vi "get_pico_rapid_data.vi"(8 "error in":errorcluster, 11 "PicoScope Acquisition Settings":T1={"Channel A Settings"={"Enabled"=TRUE, "Coupling"=1, "Range"=6, "Analogue Offset"=0.0}, "Channel B Settings"={"Enabled"=TRUE, "Coupling"=1, "Range"=6, "Analogue Offset"=0.0}, "Trigger Options"={"Trigger Enabled"=FALSE, "Trigger Source"=enum."Channel A", "Trigger Threshold (-5 to 5 V)"=0.0, "Trigger Slope"=2, "Trigger Delay (s)"=0.0, "Auto Trigger Time (ms)"=1000}, "Pico Scope Inititalization Settings"={"USB Power"=FALSE, "Use Serial Number"=FALSE, "Resolution"=0, "Serial Number"="", "Handle"=0}, "Use PicoScope?"=FALSE, "Acquisition Settings"={"Pre Trigger Time (s)"=512.0, "Post Trigger Time (s)"=512.0, "Resolution (s)"=34.36, "Four Channel Device"=FALSE, "Number of Captures"=1.0}} {"Acquisition Settings"."Number of Captures" min=1.0 step=1.0; "Acquisition Settings"."Resolution (s)" min=8e-09 max=34.36 step=8e-09 format="%#_6p"; "Acquisition Settings"."Post Trigger Time (s)" min=0.0 format="%#_6p"; "Acquisition Settings"."Pre Trigger Time (s)" min=0.0 format="%#_6p"; "Pico Scope Inititalization Settings"."Resolution" items=["8-bit", "12-bit", "14-bit", "15-bit (max. 2 ch.)", "16-bit (max. 1 ch.)"]; "Trigger Options"."Trigger Slope" items=["Rising"=2, "Falling"=3]; "Channel B Settings"."Range" items=["10 mV", "20 mV", "50 mV", "100 mV", "200 mV", "500 mV", "1 V", "2 V", "5 V", "10 V", "20 V", "50 V ", "100 V"]; "Channel B Settings"."Coupling" items=["AC", "DC"]; "Channel A Settings"."Range" items=["10 mV", "20 mV", "50 mV", "100 mV", "200 mV", "500 mV", "1 V", "2 V", "5 V", "10 V", "20 V", "50 V ", "100 V"]; "Channel A Settings"."Coupling" items=["AC", "DC"]}) -> (0 "error out":errorcluster, 2 "Channel B Out":dbl[][][](array[numeric]), 3 "Channel A Out":dbl[][][](array[numeric]))   [LabVIEW 2016]
uses:
  Controls/PicoScope/pico_control_panel.ctl
  Controls/PicoScope/pico_channel_settings.ctl
  Controls/PicoScope/pico_trigger.ctl
  Controls/PicoScope/pico_init_settings.ctl
panel:
  out "size(s)":i32[](array[numeric])
  out "Channel A Buffer":i16[][](array[numeric])
  out "Channel B Buffer":i16[][](array[numeric])
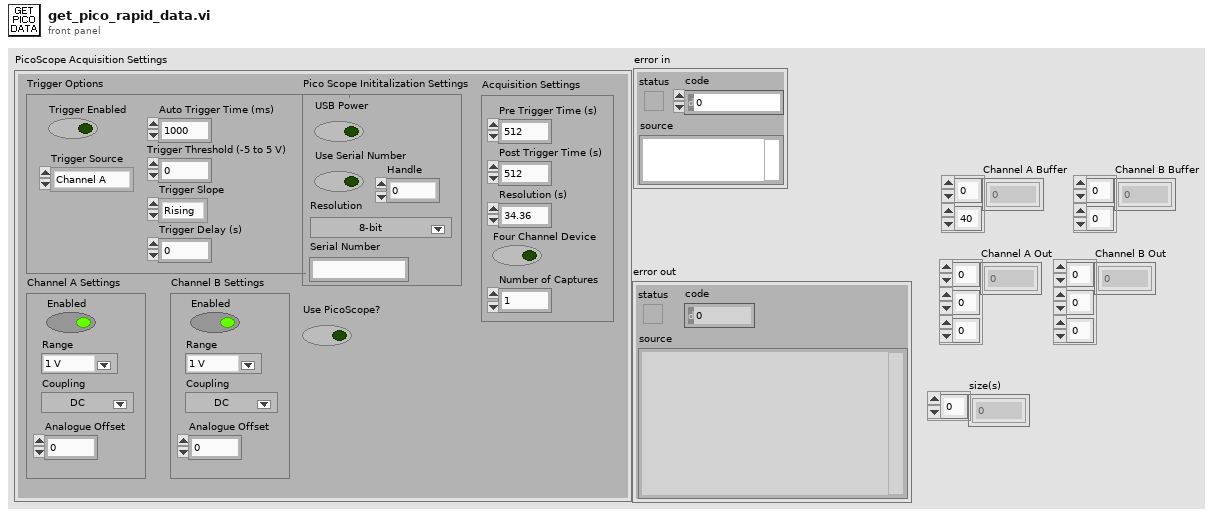
[diagram p1: front panel]
types:
  T1 = typedef "pico_control_panel.ctl" = cluster{"Channel A Settings":T2, "Channel B Settings":T2, "Trigger Options":T3, "Pico Scope Inititalization Settings":T4, "Use PicoScope?":bool, "Acquisition Settings":cluster{"Pre Trigger Time (s)":dbl, "Post Trigger Time (s)":dbl, "Resolution (s)":dbl, "Four Channel Device":bool, "Number of Captures":dbl}}
  T2 = typedef "pico_channel_settings.ctl" = cluster{"Enabled":bool, "Coupling":i16, "Range":u16, "Analogue Offset":sgl}
  T3 = typedef "pico_trigger.ctl" = cluster{"Trigger Enabled":bool, "Trigger Source":enum16{"Channel A", "Channel B", "Channel C", "Channel D", "Ext."}, "Trigger Threshold (-5 to 5 V)":dbl, "Trigger Slope":u16, "Trigger Delay (s)":dbl, "Auto Trigger Time (ms)":i16}
  T4 = typedef "pico_init_settings.ctl" = cluster{"USB Power":bool, "Use Serial Number":bool, "Resolution":i32, "Serial Number":string, "Handle":i16}
  T5 = cluster{"Pre Trigger Time (s)":dbl, "Post Trigger Time (s)":dbl, "Resolution (s)":dbl, "Four Channel Device":bool, "Number of Captures":dbl}
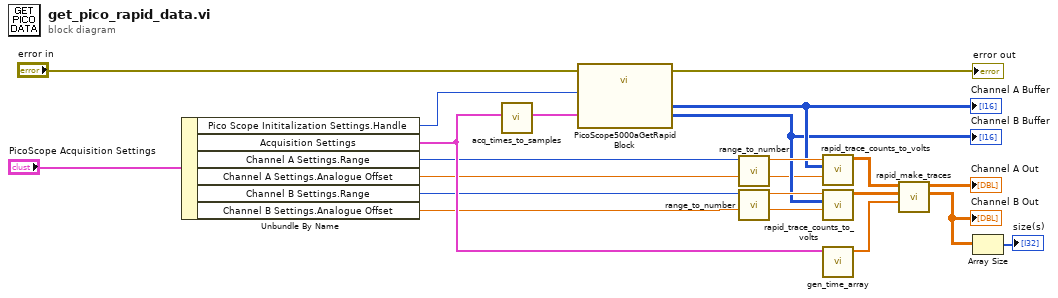
[diagram p0: block diagram]
diagram:
  n1 = Unbundle By Name("PicoScope Acquisition Settings") -> ("Pico Scope Inititalization Settings.Handle"=w5:i16, "Acquisition Settings"=w8:T5, "Channel A Settings.Range"=w4:u16, "Channel A Settings.Analogue Offset"=w3:sgl, "Channel B Settings.Range"=w2:u16, "Channel B Settings.Analogue Offset"=w1:sgl)
  n2 = call "acq_times_to_samples.vi"("Acquisition Settings"=w8) -> ("Settings to Pico"=w12:T5)  [unwired: 10 in]
  n3 = call "PicoScope5000aGetRapidBlock.vi"("error in"="error in", "handle in"=w5, "Rapid Block Acquisition Settings"=w12) -> ("Channel A Buffer"=w11:i16[][], "Channel B Buffer"=w10:i16[][], "error out"=→"error out":errorcluster)  [unwired: 7 in, 3 out]
  "Channel B Buffer" <- w10
  "Channel A Buffer" <- w11
  n4 = call "range_to_number.vi"("Channel A Settings.Range"=w4) -> ("Voltage Range"=w17:dbl)  [unwired: 10 in]
  n5 = call "range_to_number.vi"("Channel A Settings.Range"=w2) -> ("Voltage Range"=w16:dbl)  [unwired: 10 in]
  n6 = call "rapid_trace_counts_to_volts.vi"("Offset"=w3, "Channel A Buffer"=w11, "Voltage Range"=w17) -> ("Voltage Out"=w14:dbl[][])  [unwired: 8 in]
  n7 = call "rapid_trace_counts_to_volts.vi"("Offset"=w1, "Channel A Buffer"=w10, "Voltage Range"=w16) -> ("Voltage Out"=w15:dbl[][])  [unwired: 8 in]
  n8 = call "gen_time_array.vi"("Acquisition Settings"=w8) -> ("Time Out"=w13:dbl[])  [unwired: 10 in]
  n9 = call "rapid_make_traces.vi"("Time"=w13, "Channel B"=w15, "Channel A"=w14) -> ("Channel B Out"=w7:dbl[][][], "Channel A Out"=→"Channel A Out":dbl[][][])  [unwired: 7 in]
  "Channel B Out" <- w7
  n10 = Array Size(array=w7) -> (size(s)=→"size(s)":i32[])
